vi "Format data to plot_IIT.vi"(8 "Data Array 2":dbl[][](array[numeric]), 10 "Device Area (cm^2)":dbl=0.12, 11 "Data Array":dbl[][](array[numeric])) -> (3 "JV Curve":cluster{"Y":dbl[], "Y":dbl[]}[](graph))   [LabVIEW 2011]
panel:
  in  "Tab Control 4":enum32{"Page 1"}(tab)
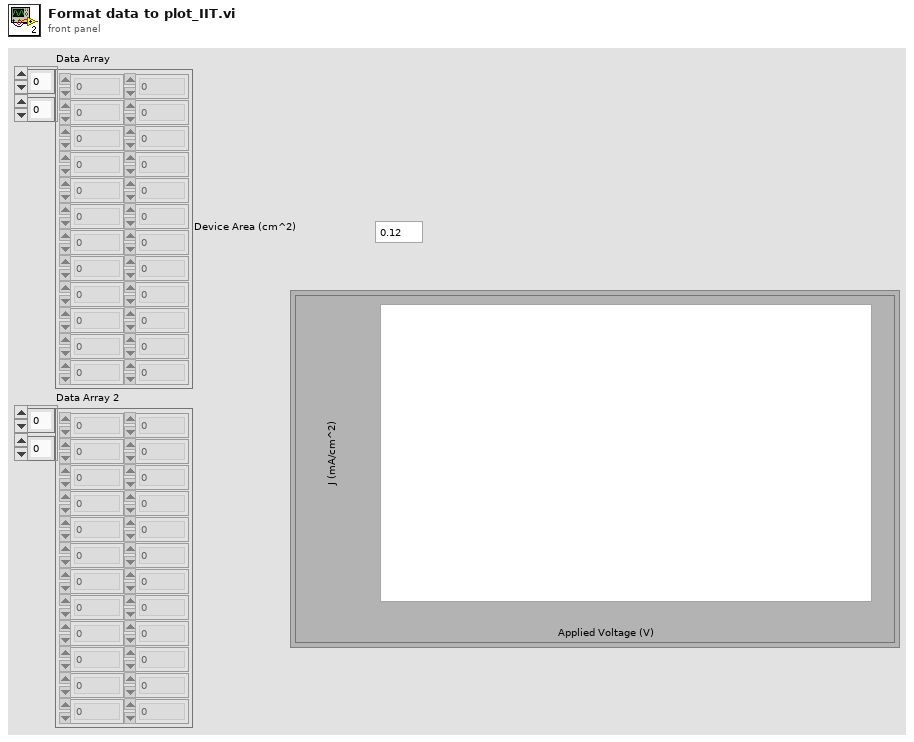
[diagram p1: front panel]
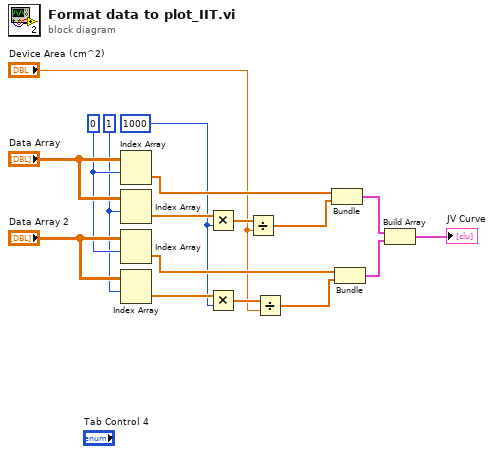
[diagram p0: block diagram]
diagram:
  w4 = 1000
  w10 = 1
  w11 = 0
  n1 = Index Array(array="Data Array", index (row)=w11) -> (element=w15:dbl[])  [unwired: 1 in]
  n2 = Index Array(array="Data Array", index (row)=w10) -> (element=w7:dbl[])  [unwired: 1 in]
  n3 = Index Array(array="Data Array 2", index (row)=w11) -> (element=w14:dbl[])  [unwired: 1 in]
  n4 = Index Array(array="Data Array 2", index (row)=w10) -> (element=w8:dbl[])  [unwired: 1 in]
  n5 = Multiply(x=w7, y=w4) -> (x*y=w6:dbl[])
  n6 = Multiply(x=w8, y=w4) -> (x*y=w5:dbl[])
  n7 = Divide(x=w6, y="Device Area (cm^2)") -> (x/y=w2:dbl[])
  n8 = Divide(x=w5, y="Device Area (cm^2)") -> (x/y=w1:dbl[])
  n9 = Bundle("Data Array"=w15, w2) -> (w12:cluster{"Data Array":dbl[], dbl[]})  [unwired: 1 in]
  n10 = Bundle("Data Array 2"=w14, w1) -> (w13:cluster{"Data Array 2":dbl[], dbl[]})  [unwired: 1 in]
  n11 = Build Array(w12, w13) -> (→"JV Curve":cluster{"Data Array 2":dbl[], dbl[]}[])
